vi "get_user_defined_flag.vi"(4 "error in (no error)":errorcluster, 6 "Container State":T2, 7 "Display State In":T1) -> (0 "error out":errorcluster, 2 "Value":bool, 3 "Display State Out":T1)   [LabVIEW 2010, in "XSettings.xctl"]
uses:
  XSettings.xctl
  <vilib>/_xctls/Container State.ctl
  state.ctl
  <vilib>/_xctls/XControlSupport.lvlib
panel:
  # "Replace the Value Indicator below with an Indicator of desired type.\nDo not remove this Indicator or the others from the connector pane. \nDo not change the connector pane pattern.\nThe Value Indicator should always be the second terminal from top on the output side in the connector pane."
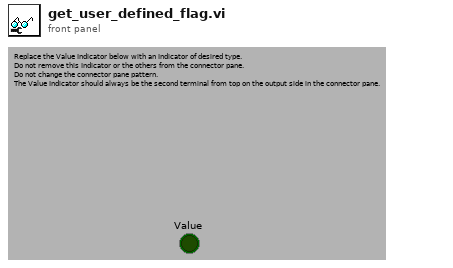
[diagram p1: front panel]
types:
  T1 = typedef "XSettings.xctl/state.ctl" = cluster{"error":errorcluster, "user-defined?":bool, "control refs":cluster{"settings combo":refnum<vi>}}
  T2 = typedef "XControlSupport.lvlib/Container State.ctl" = cluster{"Indicator?":bool, "Run Mode?":bool, " Refnum":refnum<vi>}
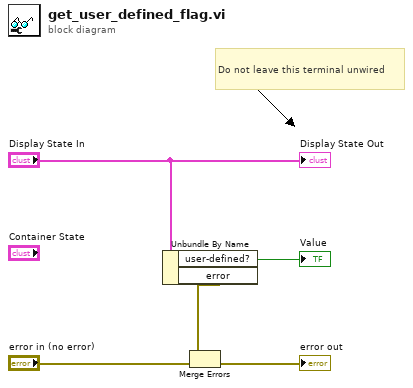
[diagram p0: block diagram]
diagram:
  # "Do not leave this terminal unwired"
  n1 = Unbundle By Name("Display State In") -> ("user-defined?"=→"Value":bool, "error"=w3:errorcluster)
  n2 = Merge Errors(w3, "error in (no error)") -> (→"error out":errorcluster)
  "Display State Out" <- "Display State In"
